vi "TiePie.Scp.ScoGetData1Ch _arraydatapoiter.vi"(0 "GenHandle":T1, 5 "pBufferCh1":dbl[](array[numeric]), 7 "qwStartIndex":u64, 9 "qwSampleCount":u64, 11 "error in (no error)":errorcluster) -> (4 "GenHandle out":T1, 6 "return type":u8, 8 "pBufferCh1 2":dbl[](array[numeric]), 15 "error out":errorcluster)   [LabVIEW 2014, in "LVTiePie.lvlib"]
uses:
  LVTiePie.lvlib
  TiePie.Gen.handle.ctl
  bin/libtiepie.dll
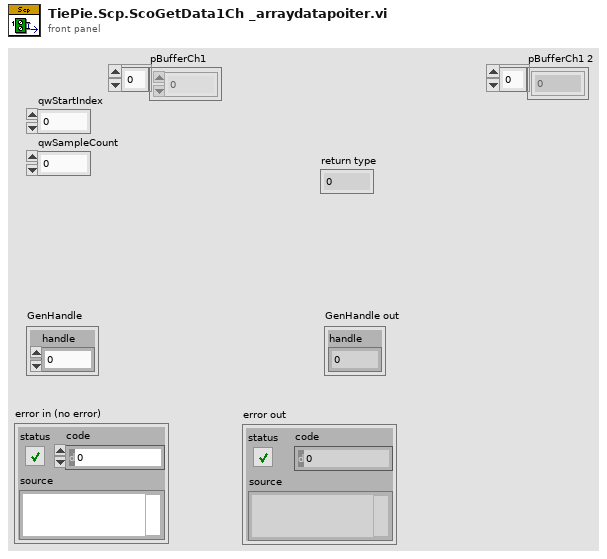
[diagram p1: front panel]
types:
  T1 = typedef "TiePie.Gen.handle.ctl" = cluster{"handle":u32}
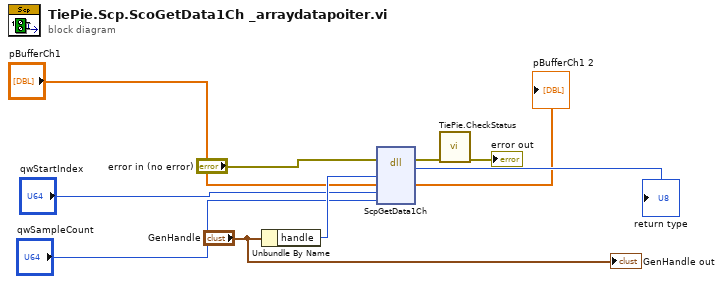
[diagram p0: block diagram]
diagram:
  n1 = Unbundle By Name("GenHandle") -> ("handle"=w9:u32)
  n2 = dll-call lib="C:/Users/mbirski/Desktop/PAN/LabVEW/Tie Pie/bin/libtiepie.dll" fn="ScpGetData1Ch"(error in="error in (no error)", "handle"=w9, "pBufferCh1"="pBufferCh1", "qwStartIndex"="qwStartIndex", "qwSampleCount"="qwSampleCount") -> (error out=w7:errorcluster, "data"=→"return type":u64, "pBufferCh1"=→"pBufferCh1 2":dbl[])  [unwired: 5 in, 1 out]
  n3 = call "TiePie.CheckStatus.vi"("error in (no error)"=w7) -> ("error out"=→"error out":errorcluster)  [unwired: 10 in]
  "GenHandle out" <- "GenHandle"
